vi "Configure Programmer Configuration Mode Parameters.vi"(0 "VISA resource name":refnum<visa-resource-name>, 1 "Unit Address (1)":u8=1, 5 "Enable Servo Action (False)":bool, 7 "Enable Synchronization (False)":bool, 9 "Action On Power Failure (0:Ramp back)":u8(ring) items=["Ramp back", "Reset", "Continue"], 11 "error in (no error)":errorcluster, 12 "Enable Fast Run (False)":bool) -> (4 "VISA resource name out":refnum<visa-resource-name>, 15 "error out":errorcluster)   [LabVIEW 2014, in "Eurotherm 35xx Series.lvlib"]
doc: "This VI configure Program Setup Configuration Mode Parameters.\n\nWarning: This VI uses Controller Configuration Mode, this interrupts working process (device will not control).\nIt is recommended that the device should be disconnected from any active process."
uses:
  <instrlib>/Eurotherm 35xx Series/Eurotherm 35xx Series.lvlib
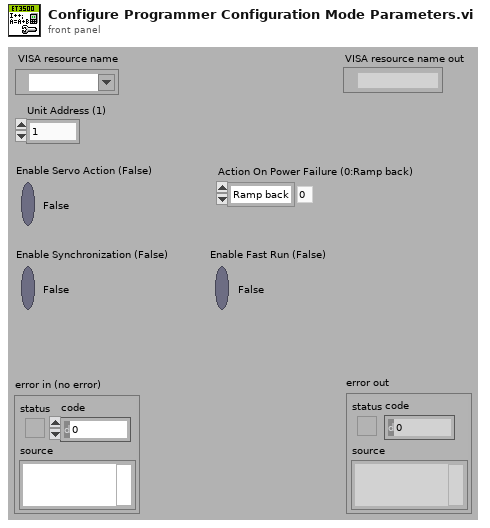
[diagram p1: front panel]
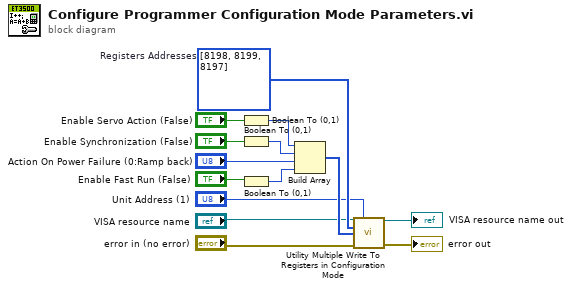
[diagram p0: block diagram]
diagram:
  w7 = u16[] [8198, 8199, 8197]  # Registers Addresses
  n1 = Boolean To (0,1)(Boolean="Enable Servo Action (False)") -> (0, 1=w3:i16)
  n2 = Boolean To (0,1)(Boolean="Enable Synchronization (False)") -> (0, 1=w10:i16)
  n3 = Boolean To (0,1)(Boolean="Enable Fast Run (False)") -> (0, 1=w1:i16)
  n4 = Build Array(w3, w10, "Action On Power Failure (0:Ramp back)", w1) -> (w8:i16[])
  n5 = call <instrlib>:"Utility Multiple Write To Registers in Configuration Mode.vi"("VISA resource name"="VISA resource name", "Unit Address (1)"="Unit Address (1)", "Registers Addresses (0)"=w7, "Data (0)"=w8, "error in (no error)"="error in (no error)") -> ("VISA resource name out"=→"VISA resource name out":refnum<visa-resource-name>, "error out"=→"error out":errorcluster)  [unwired: 9 in]
